vi "LEDHandaler.vi"(9 "Robot State":string(combo), 11 "LEDs":T1={"Traction"="Green", "Gear Ready"="Green", "Default"="Green", "Break On"=""}) -> (0 "LEDs OUT":T2, 2 "BackColor":u32(colorbox), 3 "FrontColor":u32(colorbox))   [LabVIEW 2016]
uses:
  Common Code/LED Dashboard.ctl
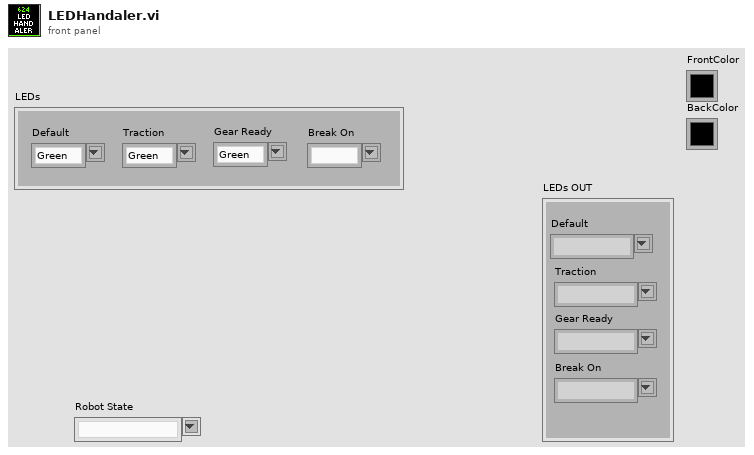
[diagram p1: front panel]
types:
  T1 = typedef "LED Dashboard.ctl" = cluster{"Traction":string, "Gear Ready":string, "Default":string, "Break On":string}
  T2 = cluster{"Default":string, "Traction":string, "Gear Ready":string, "Break On":string}
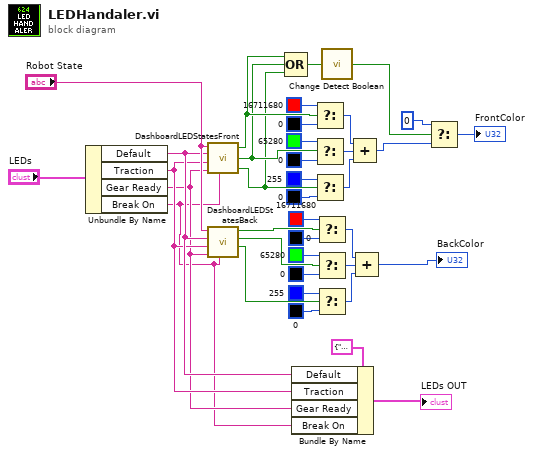
[diagram p0: block diagram]
diagram:
  n1 = Unbundle By Name("LEDs") -> ("Default"=w16:string, "Traction"=w15:string, "Gear Ready"=w14:string, "Break On"=w11:string)
  n2 = call "DashboardLEDStatesFront.vi"("State"="Robot State", "Default"=w16, "Traction"=w15, "Break On"=w11, "Gear Ready"=w14) -> ("RED"=w8:bool, "GREEN"=w7:bool, "BLUE"=w6:bool)  [unwired: 1 in]
  n3 = call "DashboardLEDStatesBack.vi"("Break On"=w11, "Gear Ready"=w14, "Traction"=w15, "Default"=w16, "State"="Robot State") -> ("BLUE"=w38:bool, "GREEN"=w37:bool, "RED"=w36:bool)  [unwired: 4 in]
  n4 = Compound Arithmetic op=OR(w8, w7, w6) -> (w9:bool)
  n5 = Bundle By Name(cluster=T2 {"Default"="", "Traction"="", "Gear Ready"="", "Break On"=""} ("LEDs IN 2"), "Default"=w16, "Traction"=w15, "Gear Ready"=w14, "Break On"=w11) -> (→"LEDs OUT":T2)
  n6 = Select(t=u32 16711680 ("FrontLED"), s=w8, f=u32 0 ("FrontLED")) -> (s? t:f=w19:u32)
  n7 = Select(t=u32 65280 ("FrontLED"), s=w7, f=u32 0 ("FrontLED")) -> (s? t:f=w20:u32)
  n8 = Select(t=u32 255 ("FrontLED"), s=w6, f=u32 0 ("FrontLED")) -> (s? t:f=w21:u32)
  n9 = Select(t=u32 16711680 ("FrontLED"), s=w36, f=u32 0 ("FrontLED")) -> (s? t:f=w35:u32)
  n10 = Select(t=u32 65280 ("FrontLED"), s=w37, f=u32 0 ("FrontLED")) -> (s? t:f=w34:u32)
  n11 = Select(t=u32 255 ("FrontLED"), s=w38, f=u32 0 ("FrontLED")) -> (s? t:f=w33:u32)
  n12 = call "Change Detect Boolean.vi"("In"=w9) -> ("Changed?"=w4:bool)
  n13 = Compound Arithmetic op=ADD(w19, w20, w21) -> (w3:u32)
  n14 = Compound Arithmetic op=ADD(w35, w34, w33) -> (→"BackColor":u32)
  n15 = Select(t=u32 0, s=w4, f=w3) -> (s? t:f=→"FrontColor":u32)
